vi "Switch_Valco_6port_subVI_BM.vi"(0 "Load (T) or Inject (F)":bool, 1 "PosA BitNum":u32=5, 2 "PosB BitNum":u32=6, 3 "BoardNum":u32=1) -> (7 "Injected":bool)   [LabVIEW 2021]
panel:
  # "PeTeR\n\nBoard: #1 (Configure using InstaCal)\n\nBit Numbers:\n0 = Sparging\n2 = Cool Trap\n4 = Drying Flow\n5 = Valve Position A\n6 = Valve Position B\n7 = Heat Trap"
  # "OSSCAR\n\nBoard: #0 (Configure using InstaCal)\n\nBit Numbers:\n0 = Sparging\n1 = Valve Position A\n2 = Valve Position B\n3 = Lights\n4 = Cool Trap\n7 = Heat Trap"
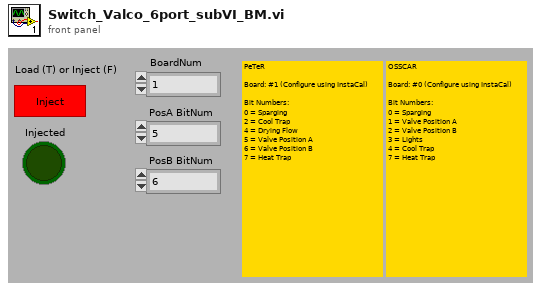
[diagram p1: front panel]
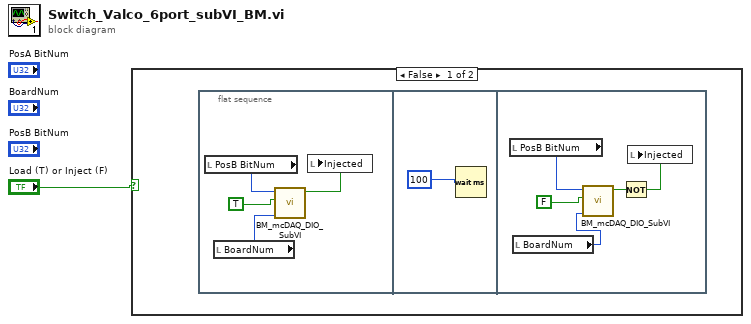
[diagram p0: block diagram]
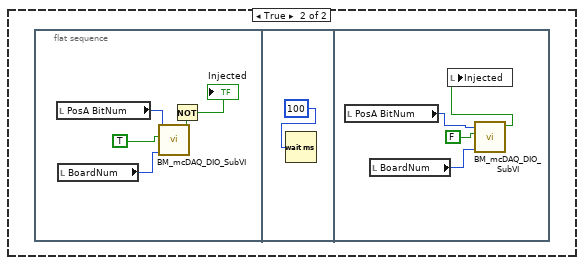
[diagram p2: hidden frame]
diagram:
  n1 = case shown="False" "Load (T) or Inject (F)" {
    frame False {
      n2 = flat-sequence {
        frame #0 {
          n3 = local read "PosB BitNum"() -> (w3:u32)
          n4 = local read "BoardNum"() -> (w2:u32)
          n5 = call "BM_mcDAQ_DIO_SubVI.vi"("BoardNum"=w2, "BitValue"=TRUE, "BitNum"=w3) -> ("Control out"=w4:bool)  [unwired: 8 in]
          n6 = local write "Injected"(w4) -> ()
        }
        frame #1 {
          n7 = Wait (ms)(milliseconds to wait=100) -> ()  [unwired: 1 out]
        }
        frame #2 {
          n8 = local read "PosB BitNum"() -> (w8:u32)
          n9 = local read "BoardNum"() -> (w7:u32)
          n10 = call "BM_mcDAQ_DIO_SubVI.vi"("BoardNum"=w7, "BitValue"=FALSE, "BitNum"=w8) -> ("Control out"=w10:bool)  [unwired: 8 in]
          n11 = Not(x=w10) -> (.not. x?=w9:bool)
          n12 = local write "Injected"(w9) -> ()
        }
      }
    }
    frame True {
      n13 = flat-sequence {
        frame #0 {
          n14 = local read "PosA BitNum"() -> (w12:u32)
          n15 = local read "BoardNum"() -> (w13:u32)
          n16 = call "BM_mcDAQ_DIO_SubVI.vi"("BoardNum"=w13, "BitValue"=TRUE, "BitNum"=w12) -> ("Control out"=w15:bool)  [unwired: 8 in]
          n17 = Not(x=w15) -> (.not. x?=→"Injected":bool)
        }
        frame #1 {
          n18 = Wait (ms)(milliseconds to wait=100) -> ()  [unwired: 1 out]
        }
        frame #2 {
          n19 = local read "PosA BitNum"() -> (w18:u32)
          n20 = local read "BoardNum"() -> (w19:u32)
          n21 = call "BM_mcDAQ_DIO_SubVI.vi"("BoardNum"=w19, "BitValue"=FALSE, "BitNum"=w18) -> ("Control out"=w20:bool)  [unwired: 8 in]
          n22 = local write "Injected"(w20) -> ()
        }
      }
    }
  }
